vi "quad.vi"() -> ()   [LabVIEW 2012]
panel:
  out "String":string
  out "r2":dbl
  out "r1":dbl
  in  "c":dbl
  in  "a":dbl
  in  "b":dbl
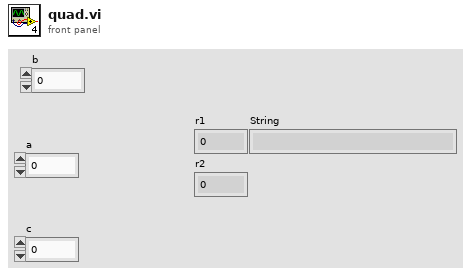
[diagram p1: front panel]
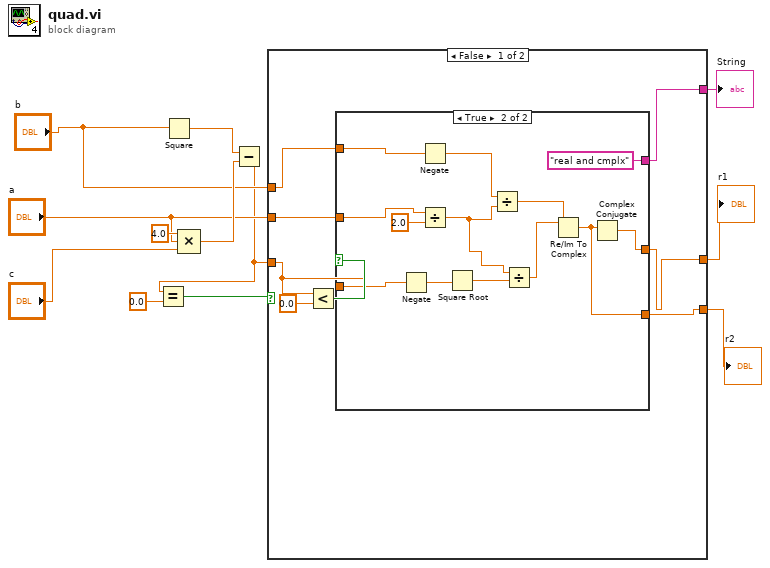
[diagram p0: block diagram]
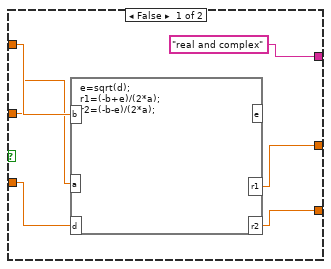
[diagram p2: hidden frame]
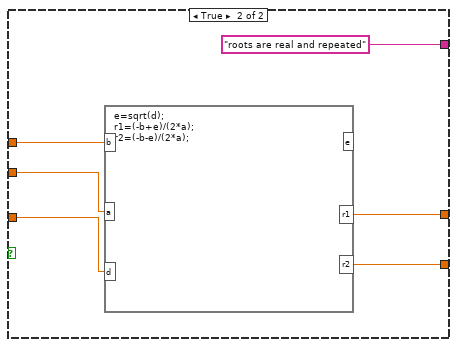
[diagram p3: hidden frame]
diagram:
  n1 = Square(x="b") -> (x^2=w10:dbl)
  n2 = Compound Arithmetic op=MULTIPLY(4.0 ("value"), "a", "c") -> (w9:dbl)
  n3 = Subtract(x=w10, y=w9) -> (x-y=w4:dbl)
  n4 = Equal?(x=w4, y=0.0) -> (x = y?=w7:bool)
  n5 = case shown="False" w7 {
    tunnel: "b" -> [w18 w45]
    tunnel: "a" -> [w17 w44]
    tunnel: w4 -> [w16 w43]
    tunnel: [w15 w42] -> w3
    tunnel: [w14 w41] -> w2
    tunnel: [w13 "roots are real and repeated"] -> w1
    frame False {
      n6 = Less?(x=w16, y=0.0) -> (x < y?=w19:bool)
      n7 = case shown="True" w19 {
        tunnel: w18 -> [w26 w39]
        tunnel: w17 -> [w25 w37]
        tunnel: w16 -> [w24 w36]
        tunnel: [w23 w29] -> w15
        tunnel: [w22 w28] -> w14
        tunnel: ["real and complex" "real and cmplx"] -> w13
        frame False {
          n8 = formula code="e=sqrt(d);\nr1=(-b+e)/(2*a);\nr2=(-b-e)/(2*a);"("b"=w26, "a"=w25, "d"=w24) -> ("r1"=w23:dbl, "r2"=w22:dbl)  [unwired: 1 out]
        }
        frame True {
          n9 = Negate(x=w36) -> (-x=w35:dbl)
          n10 = Negate(x=w39) -> (-x=w32:dbl)
          n11 = Divide(x=w37, y=2.0) -> (x/y=w33:dbl)
          n12 = Square Root(x=w35) -> (sqrt(x)=w34:dbl)
          n13 = Divide(x=w32, y=w33) -> (x/y=w31:dbl)
          n14 = Divide(x=w33, y=w34) -> (x/y=w30:dbl)
          n15 = Re/Im To Complex(1:w31, 2:w30) -> (0:w28:cdb)
          n16 = Complex Conjugate(1:w28) -> (0:w29:cdb)
        }
      }
    }
    frame True {
      n17 = formula code="e=sqrt(d);\nr1=(-b+e)/(2*a);\nr2=(-b-e)/(2*a);"("b"=w45, "a"=w44, "d"=w43) -> ("r1"=w42:dbl, "r2"=w41:dbl)  [unwired: 1 out]
    }
  }
  "r1" <- w3
  "r2" <- w2
  "String" <- w1
